vi "Basic Sine RX - Template.vi"() -> ()   [LabVIEW 2013]
uses:
  <instrlib>/niUSRP/niUSRP Fetch Rx Data (CDB WDT).vi
  <vilib>/express/express analysis/Spectral/Block/exnSpectralBlock spectral measurements RMS poly.vi
  <vilib>/express/express analysis/Spectral/Block/exnSpectralBlock spectral measurements RMS WFM.vi
  <vilib>/express/express analysis/Spectral/XNode/ExpressSpectralMeasurementsBlockNode.xnode
panel:
  out "Spectrum":cluster{"f0":dbl, "df":dbl, "magnitude":dbl[]}(graph)={"f0"=0.0, "df"=2.0, "magnitude"=array[50000 elements]}
  out "error out":errorcluster
  out "coerced gain":dbl format="%#_6f"
  out "coerced IQ rate":dbl=200000.0 format="%#_6p"
  out "coerced carrier frequency":dbl=2400000000.0 format="%#_6p"
  out "Waveform":waveform(dbl)[](graph)
  in  "number of samples":i64=100000
  in  "stop":bool
  in  "device names":refnum<k15>="192.168.10.2"
  in  "active antenna":string="RX2"
  in  "gain":dbl format="%#_6f"
  in  "carrier frequency":dbl=2400000000.0 format="%#_6p"
  in  "IQ rate":dbl=200000.0 format="%#_6p"
  # "USRP Receiver"
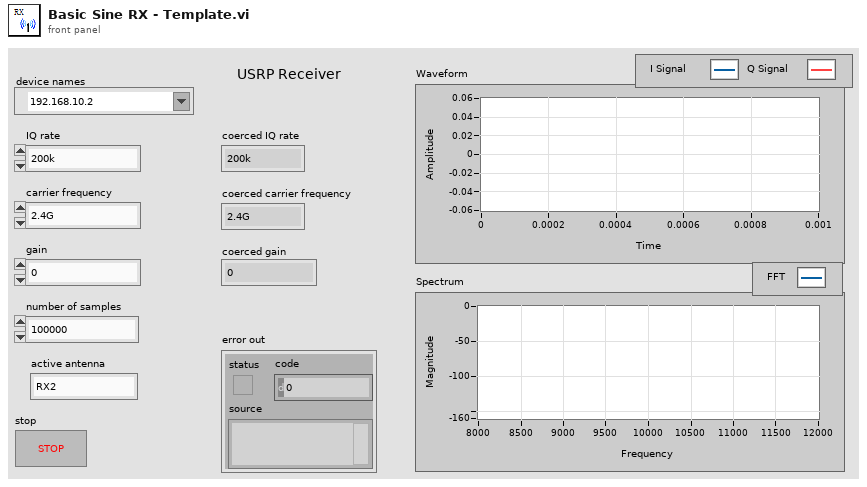
[diagram p1: front panel]
types:
  T1 = cluster{"averaging mode":u16, "weighting mode":u16, "number of averages":u32}
  T2 = cluster{"dB On (F)":bool, "unwrap phase (F)":bool, "convert to degree (F)":bool}
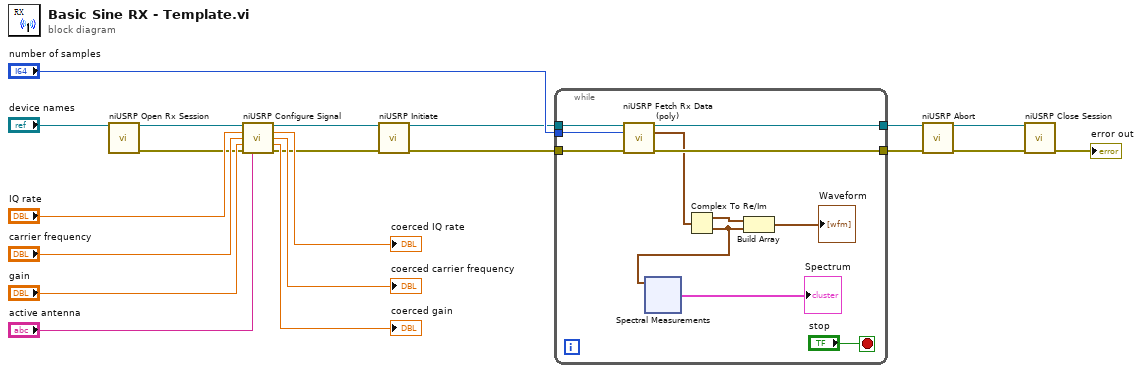
[diagram p0: block diagram]
diagram:
  n1 = call <instrlib>:"niUSRP Open Rx Session.vi"("device names"="device names") -> ("session handle out"=w17:refnum<k15>, "error out"=w8:errorcluster)  [unwired: 13 in]
  n2 = call <instrlib>:"niUSRP Configure Signal.vi"("session handle"=w17, "IQ rate"="IQ rate", "carrier frequency"="carrier frequency", "gain"="gain", "error in (no error)"=w8, "active antenna"="active antenna") -> ("session handle out"=w16:refnum<k15>, "coerced IQ rate"=→"coerced IQ rate":dbl, "coerced carrier frequency"=→"coerced carrier frequency":dbl, "coerced gain"=→"coerced gain":dbl, "error out"=w7:errorcluster)  [unwired: 5 in]
  n3 = call <instrlib>:"niUSRP Initiate.vi"("session handle"=w16, "error in (no error)"=w7) -> ("session handle out"=w18:refnum<k15>, "error out"=w6:errorcluster)  [unwired: 12 in]
  n4 = while {
    tunnel: "number of samples" -> [w29]
    tunnel: w18 -> [w30]
    tunnel: w6 -> [w28]
    tunnel: [w27] -> w5
    tunnel: [w26] -> w4
    stop <- "stop" stop-if-true
    n5 = call-poly <instrlib>:"niUSRP Fetch Rx Data (poly).vi"("session handle"=w30, "number of samples"=w29, "error in (no error)"=w28) -> ("session handle out"=w26:refnum<k15>, "data"=w23:waveform(cdb), "error out"=w27:errorcluster)  [unwired: 9 in, 1 out]
    n6 = Complex To Re/Im(x + iy=w23) -> (x=w24:waveform(dbl), y=w22:waveform(dbl))
    n7 = xnode "Spectral Measurements"("Signals"=w22) -> ("Measurement Output"=→"Spectrum":cluster{"f0":dbl, "df":dbl, "magnitude":dbl[]})  [unwired: 1 in, 2 out]
    n8 = Build Array "Build Array"(w24, w22) -> (→"Waveform":waveform(dbl)[])
  }
  n9 = call <instrlib>:"niUSRP Abort.vi"("session handle"=w4, "error in (no error)"=w5) -> ("session handle out"=w3:refnum<k15>, "error out"=w2:errorcluster)  [unwired: 12 in]
  n10 = call <instrlib>:"niUSRP Close Session.vi"("session handle"=w3, "error in (no error)"=w2) -> ("error out"=→"error out":errorcluster)  [unwired: 13 in]
